vi "Parse Control.vi"() -> ()   [LabVIEW 2016]
uses:
  <vilib>/Utility/traverseref.llb/TRef TravTarget.ctl
  <vilib>/Utility/Data Type/Type Definitions/Data Type.ctl
  <vilib>/Utility/traverseref.llb/VI Scripting - Traverse.lvlib
  <vilib>/Utility/Data Type/NI_Data Type.lvlib
panel:
  out "# of Refs":i32
  out "References":refnum<vi>[](array[refnum])
  in  "Path":path
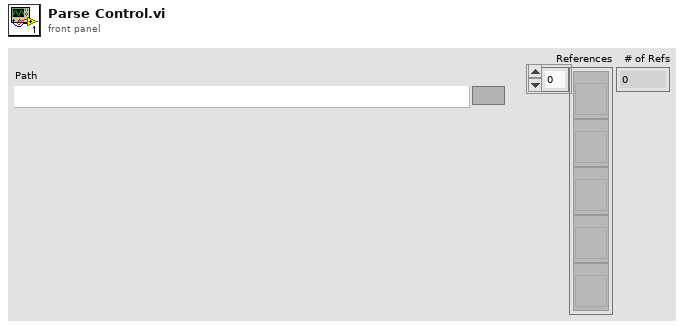
[diagram p1: front panel]
types:
  T1 = typedef "NI_Data Type.lvlib/Data Type.ctl" = enum8{"Invalid Type", "Void", "I8", "I16", "I32", "I64", "U8", "U16", "U32", "U64", "Single Float", "Double Float", "Extended Float", "Single Complex", "Double Complex", "Extended Complex", "Enum U8", "Enum U16", "Enum U32", "Enum U64", "Single Float With Unit", "Double Float With Unit", "Extended Float With Unit", "Single Complex with Unit", "Double Complex with Unit", "Extended Complex with Unit", "Boolean", "String", "Path", "Picture", "Tag", "Array", "Cluster", "Variant", "LV Variant", "Waveform", "Timestamp", "Digital Waveform", "Digital Data", "ExpressData", "Refnum", "External Data", "VI", "Poly VI", "LabVIEW Class Instance", "Fixed Point"}
  T2 = enum32{"invalid VI type", "Standard VI", "Control VI", "Global VI", "Polymorphic VI", "Configuration VI", "SubSystem", "Facade VI", "Method VI", "Statechart Diagram VI"}
  T3 = typedef "TRef TravTarget.ctl" = enum16{"FP", "BD", "Other"}
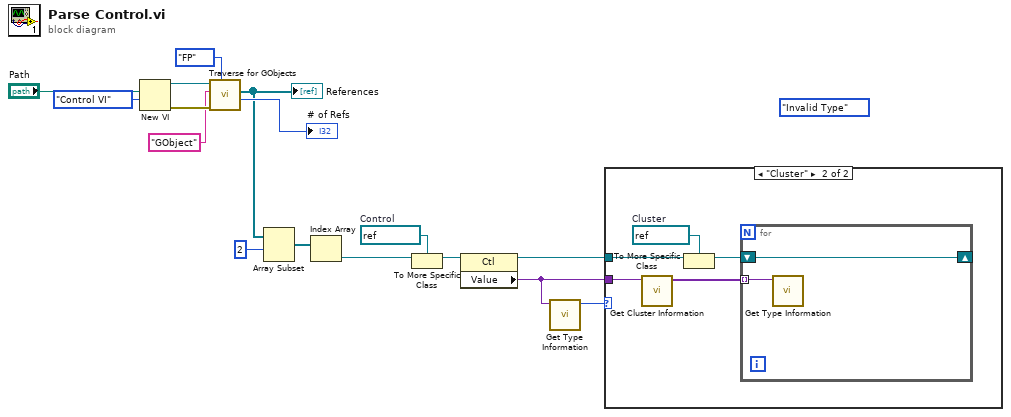
[diagram p0: block diagram]
diagram:
  (unwired) Data_Type."Invalid Type" ("Type")
  w7 = refnum<vi> refnum  # Control
  n1 = New VI(9:T2."Control VI" ("vi type (standard vi)"), 10:"Path") -> (0:w14:errorcluster, 3:w15:refnum<vi>)  [unwired: 5 in]
  n2 = call <vilib>:"Traverse for GObjects.vi"("Traverse Target"=TRef_TravTarget."FP", "error in (no error)"=w14, "Class Name"="GObject", "VI Refnum"=w15) -> ("# of Refs"=→"# of Refs":i32, "References"=w9:refnum<vi>[])  [unwired: 4 in, 2 out]
  "References" <- w9
  n3 = Array Subset(array=w9, index=2) -> (w5:refnum<vi>[])  [unwired: 1 in]
  n4 = Index Array(array=w5) -> (element=w2:refnum<vi>)  [unwired: 1 in]
  n5 = To More Specific Class(target class=w7, reference=w2) -> (specific class reference=w6:refnum<vi>)  [unwired: 1 in, 1 out]
  n6 = property class="Ctl"(reference=w6) -> (reference out=w1:refnum<vi>, "Value"=w3:variant)  [unwired: 1 in, 1 out]
  n7 = call <vilib>:"Get Type Information.vi"("Variant"=w3) -> ("Type"=w4:T1)  [unwired: 6 in, 4 out]
  n8 = case shown="\"Cluster\"" w4 {
    tunnel: w3 -> [_ w21]
    tunnel: w1 -> [_ w18]
    frame "Invalid Type", Default {
    }
    frame "Cluster" {
      w19 = refnum<vi> refnum  # Cluster
      n9 = call <vilib>:"Get Cluster Information.vi"("Variant"=w21) -> ("Cluster Elements"=w20:variant[])  [unwired: 9 in, 1 out]
      n10 = To More Specific Class(target class=w19, reference=w18) -> (specific class reference=w17:refnum<vi>)  [unwired: 1 in, 1 out]
      n11 = for {
        tunnel: w20 -> [w23] mode=indexing
        shift-right: [w22] -> _
        shift-left: w17 -> [w22]
        n12 = call <vilib>:"Get Type Information.vi"("Variant"=w23) -> ()  [unwired: 6 in, 5 out]
      }
    }
  }
